vi "Get DDG Lite Global Control Byte.vi"(8 "error in (no error)":errorcluster, 11 "control":string) -> (0 "error out":errorcluster, 2 "function return":u32, 3 "control out":string)   [LabVIEW 2014, in "atmcd32d.lvlib"]
doc: "unsigned int WINAPI GetDDGLiteGlobalControlByte(unsigned char * control);"
uses:
  atmcd32d.lvlib
  atmcd32d.dll
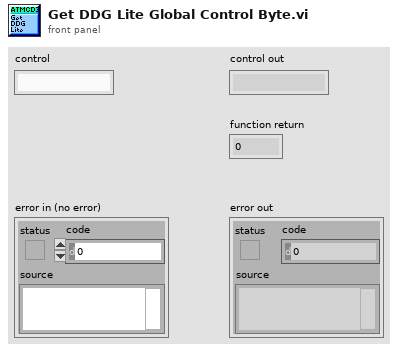
[diagram p1: front panel]
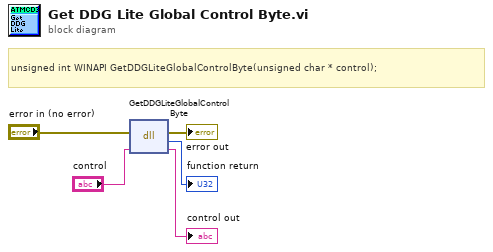
[diagram p0: block diagram]
diagram:
  # "unsigned int WINAPI GetDDGLiteGlobalControlByte(unsigned char * control);"
  n1 = dll-call lib="C:/Users/Bakir/Documents/Lambda2-Testing/lib/Andorlib/atmcd32d.*" fn="GetDDGLiteGlobalControlByte"(error in="error in (no error)", "control"="control") -> (error out=→"error out":errorcluster, →"function return":u32, "control"=→"control out":string)  [unwired: 2 in, 1 out]
